vi "Main.vi"() -> ()   [LabVIEW 2014]
doc: "This template is for the Queued Message Handler design pattern.\n\nThe Event Handling Loop generates messages based on user interface actions.\n\nThe Message Handling Loop processes messages generated by the Event Handling Loop, or by other messages. The messages are string values, so new messages can be added easily to the Message Cases case structure in the Message Handling Loop. Each message cluster can also provide an optional value for Message Data, which is a variant that can be converted to whatever message-specific data is required."
uses:
  Support/Type Definitions/UI Data.ctl
  support/Message Queue/Message Queue.lvlib
  Support/User Event - EHL Stop/User Event - EHL Stop.lvlib
  Support/Message Queue/Enqueue Message (Single).vi
  <vilib>/ErrorRing/Error Ring.xnode
  Model/Model.lvlib
  PLC/PLC.lvlib
  Support/Status Logger/Status Log.ctl
  <vilib>/Utility/error.llb/Error Cluster From Error Code.vi
  Support/Global names.vi
panel:
  out "Power status":bool
  in  "Abort":bool
  in  "Stop Line":bool
  in  "Start Line":bool
  out "Status":string
  in  "Tab Control":enum32{"Simulation"}(tab)
  in  "Power switch":bool
  in  "Positon":dbl(slide) scale=0.0..20.0
  in  "Dispose":bool
  in  "Pump":bool
  in  "Flow [l/s]":dbl=10.0
  in  "Exit":bool
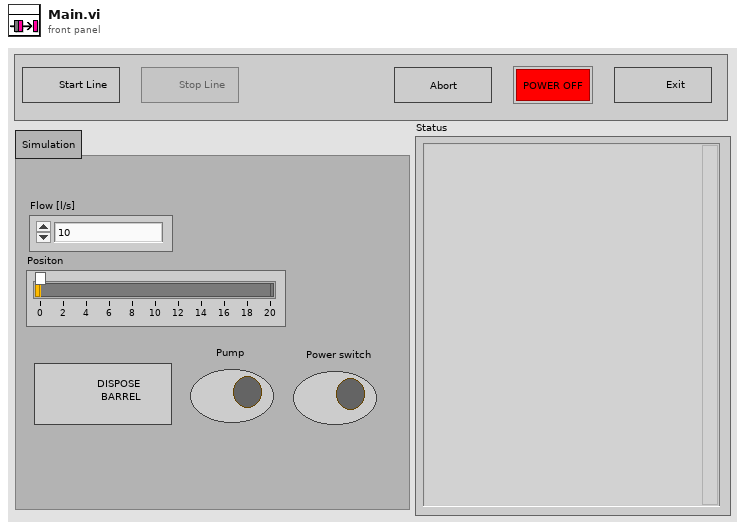
[diagram p1: front panel]
types:
  T1 = typedef "Status Log.ctl" = enum16{"Close file", "Open Status file", "Add Status", "Show Status File"}
  T2 = typedef "UI Data.ctl" = cluster{"Start Line Ref":refnum<vi>, "Stop Line Ref":refnum<vi>, "Data Display Ref":refnum<vi>, "Exit Button Ref":refnum<vi>, "Pump Ref":refnum<vi>, "Dispose Ref":refnum<vi>, "Flow Ref":refnum<vi>, "Position Ref":refnum<vi>, "Tab Ref":refnum<vi>, "Abort":refnum<vi>, "Power status":refnum<vi>, "Power switch":refnum<vi>}
  T3 = typedef "Notifiers.lvlib/Notifiers.ctl" = cluster{"PLC":refnum<notifier>, "Model":refnum<notifier>}
  T4 = typedef "Message Queue.lvlib/All Message Queues.ctl" = cluster{"UI":refnum<queue>, "Model":refnum<queue>, "PLC":refnum<queue>}
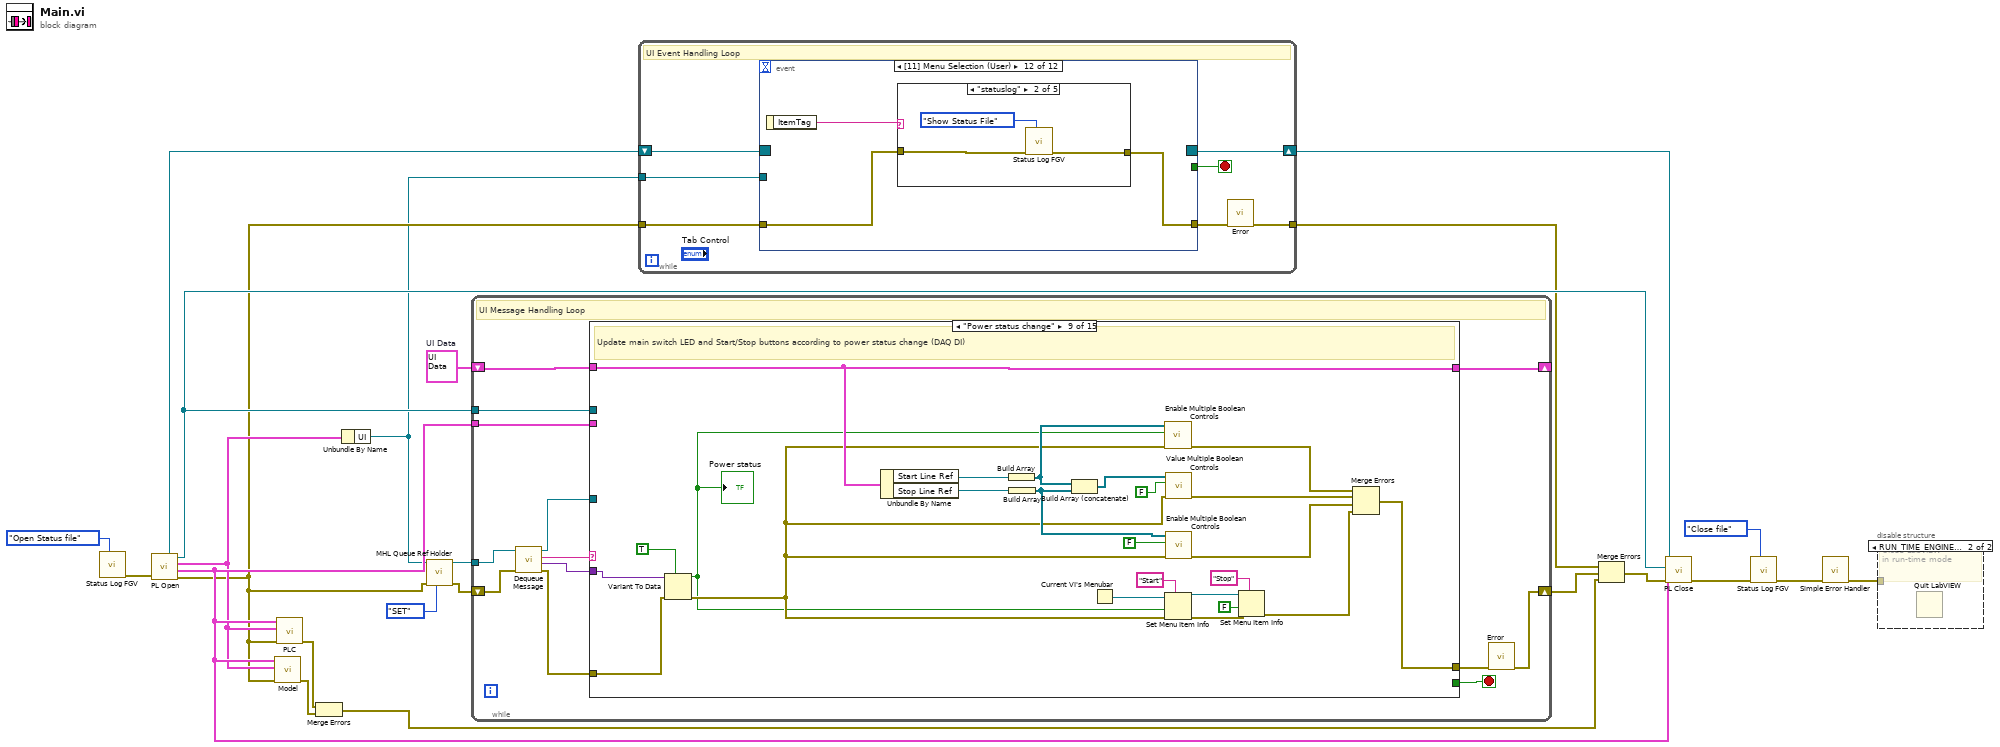
[diagram p0: block diagram]
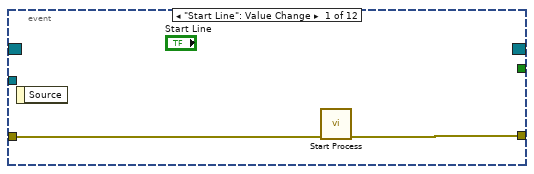
[diagram p2: hidden frame]
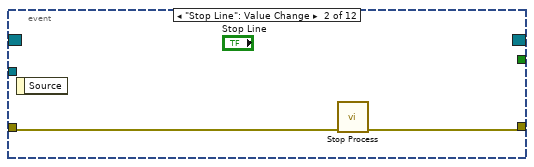
[diagram p3: hidden frame]
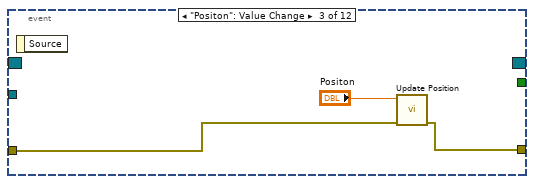
[diagram p4: hidden frame]
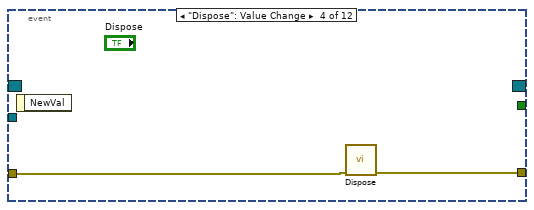
[diagram p5: hidden frame]
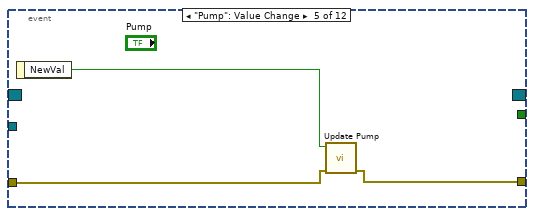
[diagram p6: hidden frame]
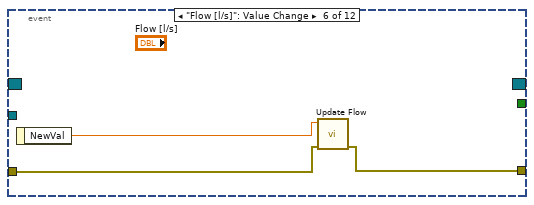
[diagram p7: hidden frame]
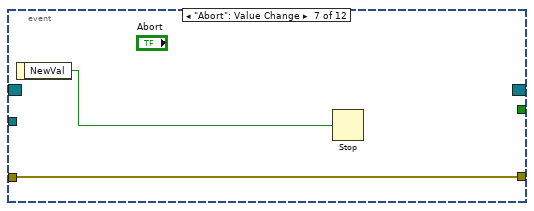
[diagram p8: hidden frame]
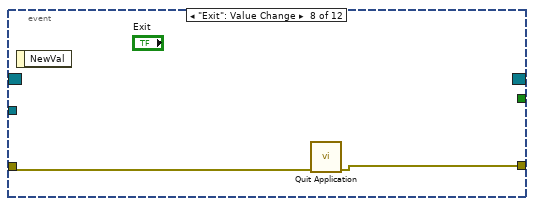
[diagram p9: hidden frame]
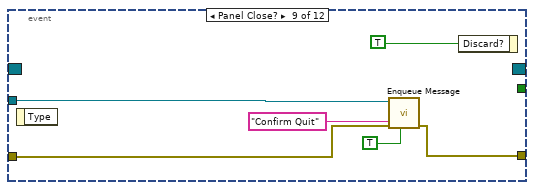
[diagram p10: hidden frame]
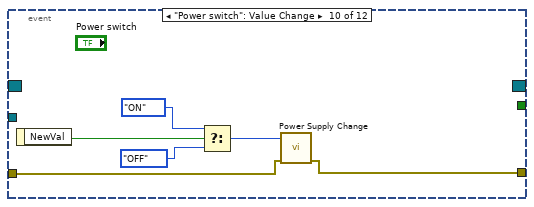
[diagram p11: hidden frame]
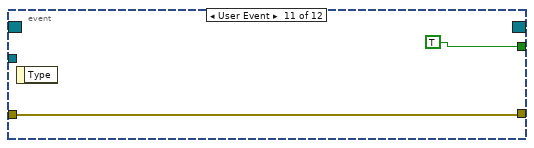
[diagram p12: hidden frame]
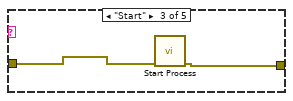
[diagram p14: hidden frame]
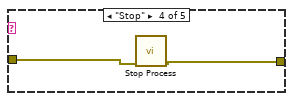
[diagram p15: hidden frame]
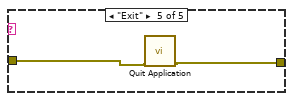
[diagram p16: hidden frame]
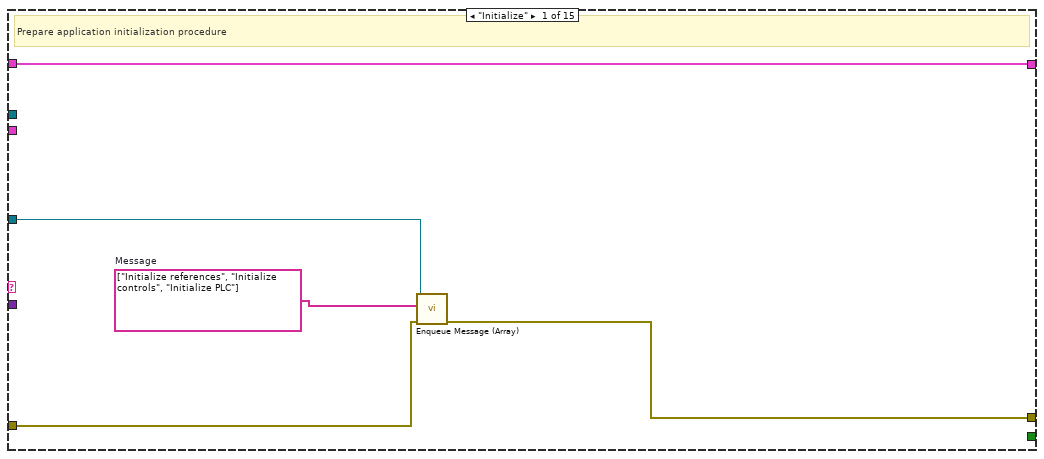
[diagram p18: hidden frame]
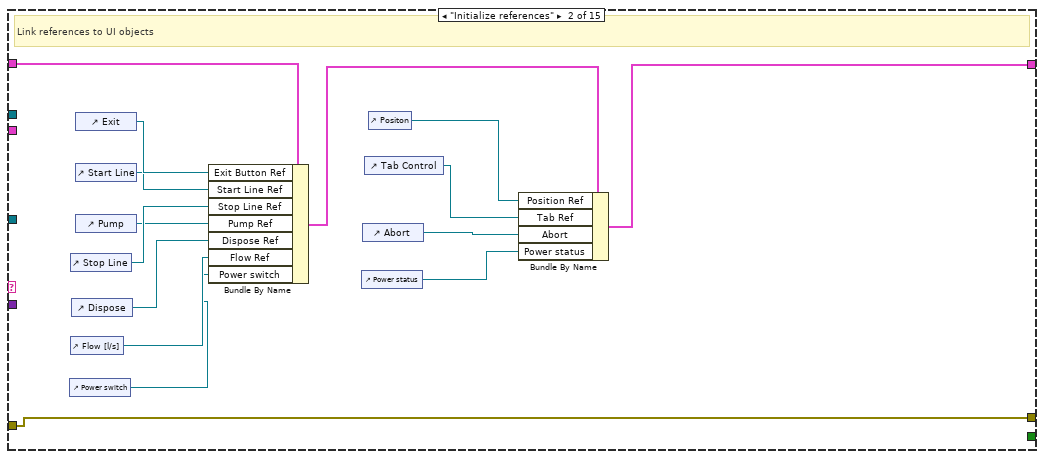
[diagram p19: hidden frame]
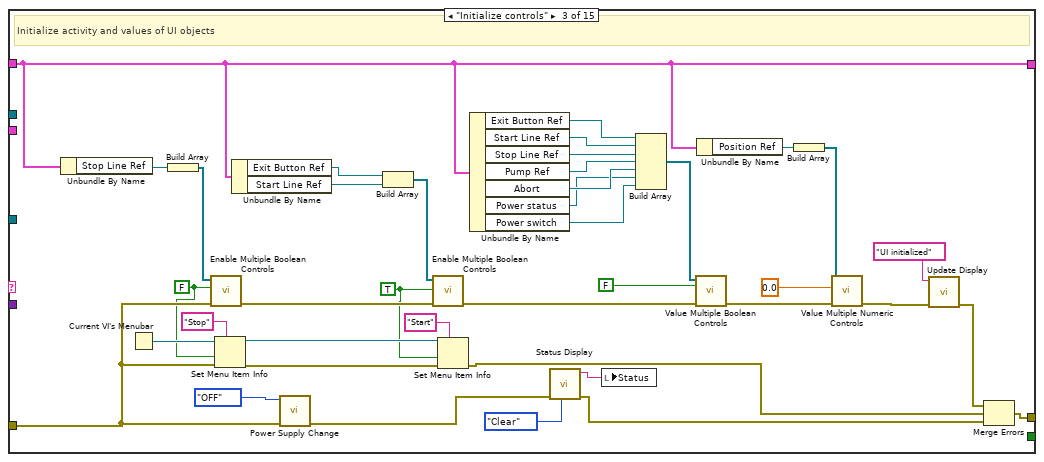
[diagram p20: hidden frame]
diagram:
  w22 = T2 {"Start Line Ref"=refnum, "Stop Line Ref"=refnum, "Data Display Ref"=refnum, "Exit Button Ref"=refnum, "Pump Ref"=refnum, "Dispose Ref"=refnum, "Flow Ref"=refnum, "Position Ref"=refnum, "Tab Ref"=refnum, "Abort"=refnum, "Power status"=refnum, "Power switch"=refnum}  # UI Data
  n1 = call "Status Log FGV.vi"("Action"=Status_Log."Open Status file") -> ("error out"=w17:errorcluster)  [unwired: 10 in]
  n2 = call "PL Open.vi"("error in"=w17) -> ("error out"=w4:errorcluster, "Notifiers"=w10:T3, "Queues"=w9:T4, "User Event"=w20:refnum<user-event>, "Event Registration Refnum"=w12:refnum<event-registration>)  [unwired: 6 in]
  n3 = call "Model.vi"("error in"=w4, "Queues"=w9, "Notifiers"=w10) -> ("error out"=w7:errorcluster)  [unwired: 8 in]
  n4 = call "PLC.vi"("error in"=w4, "Message Queues"=w9, "Notifiers"=w10) -> ("error out"=w8:errorcluster)  [unwired: 8 in]
  n5 = Merge Errors(w8, w7) -> (w6:errorcluster)
  n6 = Unbundle By Name(w9) -> ("UI"=w1:refnum<queue>)
  n7 = call "MHL Queue Ref Holder.vi"("Action"=enum16{"GET", "SET"}."SET", "error in"=w4, "Message Queue In"=w1) -> ("error out"=w3:errorcluster, "Input Message Queue"=w5:refnum<queue>)  [unwired: 7 in]
  n8 = while {
    shift-right: [w35] -> _
    shift-left: w22 -> [w36]
    tunnel: w20 -> [w33]
    tunnel: w10 -> [w29]
    shift-right: [w25] -> w16
    shift-left: w3 -> [w32]
    tunnel: w5 -> [w27]
    stop <- w34 stop-if-true
    # "UI Message Handling Loop"
    n9 = call "Dequeue Message.vi"("error in (no error)"=w32, "Message Queue"=w27) -> ("error out"=w31:errorcluster, "Message Data"=w28:variant, "Message"=w24:string, "dup Message Queue"=w30:refnum<queue>)  [unwired: 6 in]
    n10 = case "Message Cases" shown="\"Power status change\"" w24 {
      selector: w24 -> [_ _ _ _ _ _ _ _ _ _ _ _ _ _ w252]
      tunnel: w30 -> [w38 _ _ _ _ _ _ _ _ _ w198 w204 w240 _ _]
      tunnel: w31 -> [w39 w45 w65 w96 w112 w130 w143 w160 w188 w190 w199 w206 w223 w247 _]
      tunnel: [w37 w45 w74 w97 w111 w132 w145 w161 w182 w189 w196 w203 w227 w241 w251] -> w26
      tunnel: w36 -> [w40 w56 w82 w98 w117 w142 w151 w164 w185 w194 w200 w210 w232 w246 w253]
      tunnel: [w40 w46 w82 w98 w117 w142 w151 w164 w185 w194 w200 w210 w232 w246 w253] -> w35
      tunnel: [_ _ _ _ _ _ _ _ _ _ _ _ TRUE _ _] -> w34
      tunnel: w28 -> [_ _ _ _ _ _ w155 w158 w187 w193 _ _ w234 _ _]
      tunnel: w33 -> [_ _ _ _ _ _ _ _ _ _ _ _ w237 _ _]
      tunnel: w29 -> [_ _ _ _ _ _ _ _ _ _ _ w209 _ _ _]
      frame "Initialize" {
        w41 = string[] ["Initialize references", "Initialize controls", "Initialize PLC"]  # Message
        # "Prepare application initialization procedure"
        n11 = call "Enqueue Message (Array).vi"("error in (no error)"=w39, "Message Array"=w41, "Message Queue"=w38) -> ("error out"=w37:errorcluster)  [unwired: 7 in, 1 out]
      }
      frame "Initialize references" {
        # "Link references to UI objects"
        n12 = control-ref of="Power switch"() -> (w44:refnum<vi>)
        n13 = control-ref of="Stop Line"() -> (w53:refnum<vi>)
        n14 = control-ref of="Flow [l/s]"() -> (w50:refnum<vi>)
        n15 = control-ref of="Dispose"() -> (w51:refnum<vi>)
        n16 = control-ref of="Exit"() -> (w55:refnum<vi>)
        n17 = control-ref of="Start Line"() -> (w54:refnum<vi>)
        n18 = control-ref of="Pump"() -> (w52:refnum<vi>)
        n19 = Bundle By Name(cluster=w56, "Exit Button Ref"=w55, "Start Line Ref"=w54, "Stop Line Ref"=w53, "Pump Ref"=w52, "Dispose Ref"=w51, "Flow Ref"=w50, "Power switch"=w44) -> (w49:T2)
        n20 = control-ref of="Power status"() -> (w42:refnum<vi>)
        n21 = control-ref of="Abort"() -> (w43:refnum<vi>)
        n22 = control-ref of="Tab Control"() -> (w47:refnum<vi>)
        n23 = control-ref of="Positon"() -> (w48:refnum<vi>)
        n24 = Bundle By Name(cluster=w49, "Position Ref"=w48, "Tab Ref"=w47, "Abort"=w43, "Power status"=w42) -> (w46:T2)
      }
      frame "Initialize controls" {
        w57 = TRUE ("Enabled")
        w58 = FALSE ("Enabled")
        # "Initialize activity and values of UI objects"
        n25 = Unbundle By Name(w82) -> ("Stop Line Ref"=w95:refnum<vi>)
        n26 = Current VI's Menubar() -> (w60:refnum<k9>)
        n27 = Build Array(w95) -> (w94:refnum<vi>[])
        n28 = call "Enable Multiple Boolean Controls.vi"("error in"=w65, "Enabled"=w58, "References"=w94) -> ("error out"=w91:errorcluster)  [unwired: 8 in]
        n29 = Set Menu Item Info(7:"Stop" ("item tag"), 8:w65, 9:w58, 11:w60) -> (0:w63:errorcluster, 3:w59:refnum<k9>)  [unwired: 3 in]
        n30 = Unbundle By Name(w82) -> ("Exit Button Ref"=w93:refnum<vi>, "Start Line Ref"=w92:refnum<vi>)
        n31 = call "Power Supply Change.vi"("error in"=w65, "Power status"=enum16{"OFF", "ON"}."OFF") -> ("error out"=w71:errorcluster)  [unwired: 9 in]
        n32 = Build Array(w93, w92) -> (w90:refnum<vi>[])
        n33 = call "Enable Multiple Boolean Controls.vi"("error in"=w91, "Enabled"=w57, "References"=w90) -> ("error out"=w85:errorcluster)  [unwired: 8 in]
        n34 = Set Menu Item Info(7:"Start" ("item tag"), 8:w63, 9:w57, 11:w59) -> (0:w61:errorcluster)  [unwired: 3 in, 1 out]
        n35 = Unbundle By Name(w82) -> ("Exit Button Ref"=w89:refnum<vi>, "Start Line Ref"=w88:refnum<vi>, "Stop Line Ref"=w87:refnum<vi>, "Pump Ref"=w86:refnum<vi>, "Abort"=w77:refnum<vi>, "Power status"=w76:refnum<vi>, "Power switch"=w67:refnum<vi>)
        n36 = call "Status Display.vi"("Action"=enum16{"Update", "Clear"}."Clear", "error in"=w71) -> ("error out"=w70:errorcluster, "Status"=w68:string)  [unwired: 8 in]
        n37 = local write "Status"(w68) -> ()
        n38 = Build Array(w89, w88, w87, w86, w77, w76, w67) -> (w83:refnum<vi>[])
        n39 = call "Value Multiple Boolean Controls.vi"("error in"=w85, "Value"=FALSE ("Enabled"), "References"=w83) -> ("error out"=w81:errorcluster)  [unwired: 8 in]
        n40 = Unbundle By Name(w82) -> ("Position Ref"=w80:refnum<vi>)
        n41 = Build Array(w80) -> (w79:refnum<vi>[])
        n42 = call "Value Multiple Numeric Controls.vi"("error in"=w81, "Value"=0.0, "References"=w79) -> ("error out"=w73:errorcluster)  [unwired: 8 in]
        n43 = call "Update Display.vi"("error in"=w73, "Message string"="UI initialized") -> ("error out"=w62:errorcluster)  [unwired: 9 in]
        n44 = Merge Errors(w62, w61, w70) -> (w74:errorcluster)
      }
      frame "Initialize PLC" {
        # "Initialize Production Line Controller"
        n45 = call "Initialize.vi"("error in"=w96) -> ("error out"=w97:errorcluster)  [unwired: 10 in]
      }
      frame "Start process" {
        w103 = TRUE ("Enabled")
        w107 = FALSE ("Enabled")
        # "Starts process: start PLC, open logger file, create reports files, enable/disable UI controls and update status display"
        n46 = Unbundle By Name(w117) -> ("Exit Button Ref"=w100:refnum<vi>, "Start Line Ref"=w113:refnum<vi>, "Stop Line Ref"=w116:refnum<vi>)
        n47 = Build Array(w100, w113) -> (w118:refnum<vi>[])
        n48 = Build Array(w116) -> (w115:refnum<vi>[])
        n49 = call "Start.vi"("error in"=w112) -> ("error out"=w114:errorcluster)  [unwired: 10 in]
        n50 = call "Enable Multiple Boolean Controls.vi"("error in"=w112, "Enabled"=w103, "References"=w115) -> ("error out"=w105:errorcluster)  [unwired: 8 in]
        n51 = call "Enable Multiple Boolean Controls.vi"("error in"=w112, "Enabled"=w107, "References"=w118) -> ("error out"=w109:errorcluster)  [unwired: 8 in]
        n52 = global read "Global names.vi" "Starting"() -> (w101:string)
        n53 = Current VI's Menubar() -> (w102:refnum<k9>)
        n54 = call "Update Display.vi"("error in"=w114, "Message string"=w101) -> ("error out"=w99:errorcluster)  [unwired: 9 in]
        n55 = Set Menu Item Info(7:"Start" ("item tag"), 8:w109, 9:w107, 11:w102) -> (0:w108:errorcluster)  [unwired: 3 in, 1 out]
        n56 = Set Menu Item Info(7:"Stop" ("item tag"), 8:w105, 9:w103, 11:w102) -> (0:w104:errorcluster)  [unwired: 3 in, 1 out]
        n57 = Merge Errors(w99, w108, w104) -> (w111:errorcluster)
      }
      frame "Stop process" {
        w121 = FALSE ("Enabled")
        w122 = TRUE ("Enabled")
        # "Stops process: stop PLC, close logger file, save and close report files, enable/disable UI controls and update status display"
        n58 = Unbundle By Name(w142) -> ("Exit Button Ref"=w119:refnum<vi>, "Start Line Ref"=w135:refnum<vi>, "Stop Line Ref"=w141:refnum<vi>)
        n59 = call "Stop.vi"("error in"=w130) -> ("error out"=w137:errorcluster)  [unwired: 10 in]
        n60 = Build Array(w141) -> (w131:refnum<vi>[])
        n61 = Build Array(w119, w135) -> (w139:refnum<vi>[])
        n62 = global read "Global names.vi" "Stopping"() -> (w120:string)
        n63 = Build Array (concatenate)(w139, w131) -> (w138:refnum<vi>[])
        n64 = call "Enable Multiple Boolean Controls.vi"("error in"=w130, "Enabled"=w122, "References"=w139) -> ("error out"=w127:errorcluster)  [unwired: 8 in]
        n65 = call "Enable Multiple Boolean Controls.vi"("error in"=w130, "Enabled"=w121, "References"=w131) -> ("error out"=w134:errorcluster)  [unwired: 8 in]
        n66 = call "Value Multiple Boolean Controls.vi"("error in"=w130, "Value"=FALSE, "References"=w138) -> ("error out"=w133:errorcluster)  [unwired: 8 in]
        n67 = call "Update Display.vi"("error in"=w137, "Message string"=w120) -> ("error out"=w136:errorcluster)  [unwired: 9 in]
        n68 = Current VI's Menubar() -> (w128:refnum<k9>)
        n69 = Set Menu Item Info(7:"Start" ("item tag"), 8:w127, 9:w122, 11:w128) -> (0:w125:errorcluster, 3:w123:refnum<k9>)  [unwired: 3 in]
        n70 = Set Menu Item Info(7:"Stop" ("item tag"), 8:w125, 9:w121, 11:w123) -> (0:w124:errorcluster)  [unwired: 3 in, 1 out]
        n71 = Merge Errors(w136, w124, w134, w133) -> (w132:errorcluster)
      }
      frame "Update display" {
        # "Updates status display, status log file and word report file"
        n72 = Variant To Data(error in=w143, type="", Variant=w155) -> (data=w144:string, error out=w148:errorcluster)
        n73 = call "Status Display.vi"("Action"=enum16{"Update", "Clear"}."Update", "error in"=w148, "Status line"=w144) -> ("error out"=w146:errorcluster, "Status"=→"Status":string)  [unwired: 7 in]
        n74 = call "Status Log FGV.vi"("Action"=Status_Log."Add Status", "error in"=w148, "Status"=w144) -> ("error out"=w147:errorcluster)  [unwired: 8 in]
        n75 = property on="Status" class="Str"("Text.Scroll Position"=-1) -> ()  [unwired: 2 in, 2 out]
        n76 = Merge Errors(w143, w147, w146) -> (w145:errorcluster)
      }
      frame "Update position" {
        # "Programmatically update position of the barrel slider"
        n77 = Variant To Data(error in=w160, type=0.0 ("Value"), Variant=w158) -> (data=w156:dbl, error out=w159:errorcluster)
        n78 = Unbundle By Name(w164) -> ("Position Ref"=w163:refnum<vi>)
        n79 = Build Array(w163) -> (w162:refnum<vi>[])
        n80 = call "Value Multiple Numeric Controls.vi"("error in"=w159, "Value"=w156, "References"=w162) -> ("error out"=w161:errorcluster)  [unwired: 8 in]
      }
      frame "Power status change" {
        # "Update main switch LED and Start/Stop buttons according to power status change (DAQ DI)"
        n81 = Variant To Data(error in=w188, type=TRUE, Variant=w187) -> (data=w165:bool, error out=w169:errorcluster)
        "Power status" <- w165
        n82 = Unbundle By Name(w185) -> ("Start Line Ref"=w184:refnum<vi>, "Stop Line Ref"=w183:refnum<vi>)
        n83 = Build Array(w184) -> (w181:refnum<vi>[])
        n84 = Build Array(w183) -> (w178:refnum<vi>[])
        n85 = Build Array (concatenate)(w181, w178) -> (w180:refnum<vi>[])
        n86 = Current VI's Menubar() -> (w172:refnum<k9>)
        n87 = call "Enable Multiple Boolean Controls.vi"("error in"=w169, "Enabled"=w165, "References"=w181) -> ("error out"=w176:errorcluster)  [unwired: 8 in]
        n88 = Set Menu Item Info(7:"Start" ("item tag"), 8:w169, 9:w165, 11:w172) -> (0:w170:errorcluster, 3:w166:refnum<k9>)  [unwired: 3 in]
        n89 = call "Value Multiple Boolean Controls.vi"("error in"=w169, "Value"=FALSE, "References"=w180) -> ("error out"=w175:errorcluster)  [unwired: 8 in]
        n90 = call "Enable Multiple Boolean Controls.vi"("error in"=w169, "Enabled"=FALSE, "References"=w178) -> ("error out"=w174:errorcluster)  [unwired: 8 in]
        n91 = Set Menu Item Info(7:"Stop" ("item tag"), 8:w170, 9:FALSE ("enabled"), 11:w166) -> (0:w167:errorcluster)  [unwired: 3 in, 1 out]
        n92 = Merge Errors(w176, w175, w174, w167) -> (w182:errorcluster)
      }
      frame "Error" {
        # "Display error dialog box and quit application"
        n93 = Variant To Data(error in=w190, type=errorcluster {"status"=FALSE, "code"=0, "source"=""} ("error constant"), Variant=w193) -> (data=w191:errorcluster, error out=w189:errorcluster)
        n94 = call <vilib>:"Simple Error Handler.vi"("error in (no error)"=w191) -> ()  [unwired: 4 in, 5 out]
      }
      frame "Exit" {
        # "Start exit procedure: stop PLC, then send Exit message to PLC and go to PLC confirmation loop"
        n95 = Flush Queue(queue=w198, error in (no error)=w199) -> (error out=w195:errorcluster)  [unwired: 2 out]
        n96 = call "Exit PLC.vi"("error in"=w195) -> ("error out"=w197:errorcluster)  [unwired: 10 in]
        n97 = call "Wait on PLC Exit.vi"("error in"=w197) -> ("error out"=w196:errorcluster)  [unwired: 10 in]
      }
      frame "Wait on PLC exit" {
        # "Wait until PLC shutdown"
        n98 = Unbundle By Name(w209) -> ("PLC"=w208:refnum<notifier>)
        n99 = Wait on Notification(notifier=w208, timeout in ms (-1)=10, error in (no error)=w206) -> (notification=w202:string, timed out?=w205:bool, error out=w201:errorcluster)  [unwired: 1 in, 1 out]
        n100 = case shown="True" w205 {
          tunnel: [w211 w220] -> w203
          tunnel: w201 -> [w212 w217]
          tunnel: w204 -> [_ w218]
          tunnel: w202 -> [_ w213]
          frame True {
            # "Shutdown notification from PLC not received"
            n101 = call "Wait on PLC Exit.vi"("error in"=w212) -> ("error out"=w211:errorcluster)  [unwired: 10 in]
          }
          frame False {
            # "Shutdown notification from PLC received (handshake)"
            n102 = call "Update Display.vi"("error in"=w217, "Message string"=w213) -> ("error out"=w216:errorcluster)  [unwired: 9 in]
            n103 = call "Update Display.vi"("error in"=w216, "Message string"="Application quits" ("Message")) -> ("error out"=w215:errorcluster)  [unwired: 9 in]
            n104 = call-poly "Enqueue Message.vi"("error in (no error)"=w215, "Message"="End program", "Message Queue"=w218) -> ("error out"=w220:errorcluster)  [unwired: 7 in, 1 out]
          }
        }
      }
      frame "End program" {
        # "Shutdown MHL and send exit user event to EHL; reset UI controls"
        n105 = call "Fire User Event - EHL Stop.vi"("error in (no error)"=w223, "User Event - Stop"=w237) -> ("error out"=w222:errorcluster)  [unwired: 9 in]
        n106 = Variant To Data(error in=w223, type=errorcluster {"status"=FALSE, "code"=0, "source"=""} ("error constant"), Variant=w234) -> (data=w235:errorcluster)  [unwired: 1 out]
        n107 = Release Queue(queue=w240, force destroy? (F)=TRUE, error in (no error)=w223) -> (error out=w238:errorcluster)  [unwired: 2 out]
        n108 = call <vilib>:"Simple Error Handler.vi"("error in (no error)"=w235) -> ("error out"=w221:errorcluster)  [unwired: 4 in, 4 out]
        n109 = Merge Errors(w222, w221, w238) -> (w228:errorcluster)
        n110 = Unbundle By Name(w232) -> ("Exit Button Ref"=w231:refnum<vi>, "Abort"=w226:refnum<vi>, "Start Line Ref"=w225:refnum<vi>, "Stop Line Ref"=w224:refnum<vi>)
        n111 = Build Array(w231, w226, w225, w224) -> (w230:refnum<vi>[])
        n112 = call "Value Multiple Boolean Controls.vi"("error in"=w228, "Value"=FALSE, "References"=w230) -> ("error out"=w227:errorcluster)  [unwired: 8 in]
      }
      frame "Confirm Quit" {
        # "Confirm Quit - Message that can confirm whether or not the user wants to exit the application."
        n113 = Two Button Dialog(message="Are you sure?", 1:"Continue" ("F button name (\"Cancel\")"), 2:"Quit" ("T button name (\"OK\")")) -> (T button?=w242:bool)
        n114 = case shown="True" w242 {
          tunnel: w247 -> [w248 w250]
          tunnel: [w248 w249] -> w241
          frame False {
          }
          frame True {
            n115 = call "Quit Application.vi"("error in"=w250) -> ("error out"=w249:errorcluster)  [unwired: 10 in]
          }
        }
      }
      frame Default {
        # "Incorrect message: show error and clear error"
        n116 = xnode "Error Ring"("parameter 0"=w252) -> ("error out"=w251:errorcluster)
      }
    }
    n117 = call "Error.vi"("error in"=w26) -> ("error out"=w25:errorcluster)  [unwired: 10 in]
  }
  n118 = while {
    tunnel: w1 -> [w263]
    shift-right: [w266] -> w23
    shift-left: w12 -> [w267]
    tunnel: [w261] -> w11
    tunnel: w4 -> [w264]
    stop <- w265 stop-if-true
    # "UI Event Handling Loop"
    n119 = event shown="[11] Menu Selection (User)" {
      selector: w267 -> [_ _ _ _ _ _ _ _ _ _ _ _]
      dyn-events: [_ _ _ _ _ _ _ _ _ _ _ _] -> w266
      timeout: _ -> [_ _ _ _ _ _ _ _ _ _ _ _]
      tunnel: [_ _ _ _ _ _ _ _ _ _ TRUE ("Discard?") _] -> w265
      tunnel: w263 -> [_ _ _ _ _ _ _ _ w292 _ _ _]
      tunnel: [w268 w270 w273 w275 w278 w281 w284 w285 w291 w293 w299 w302] -> w262
      tunnel: w264 -> [w269 w271 w272 w276 w279 w282 w284 w286 w287 w294 w299 w301]
      event "Start Line": Value Change {
        n120 = event-data() -> ()  [unwired: 1 in, 1 out]
        n121 = call "Start Process.vi"("error in"=w269) -> ("error out"=w268:errorcluster)  [unwired: 10 in]
      }
      event "Stop Line": Value Change {
        n122 = event-data() -> ()  [unwired: 1 in, 1 out]
        n123 = call "Stop Process.vi"("error in"=w271) -> ("error out"=w270:errorcluster)  [unwired: 10 in]
      }
      event "Positon": Value Change {
        n124 = event-data() -> ()  [unwired: 1 in, 1 out]
        n125 = call "Update Position.vi"("error in (no error)"=w272, "Position"="Positon") -> ("error out"=w273:errorcluster)  [unwired: 9 in]
      }
      event "Dispose": Value Change {
        n126 = event-data() -> ()  [unwired: 1 in, 1 out]
        n127 = call "Dispose.vi"("error in (no error)"=w276) -> ("error out"=w275:errorcluster)  [unwired: 10 in]
      }
      event "Pump": Value Change {
        n128 = event-data() -> ("NewVal"=w277:bool)  [unwired: 1 in]
        n129 = call "Update Pump.vi"("error in (no error)"=w279, "Pump State"=w277) -> ("error out"=w278:errorcluster)  [unwired: 9 in]
      }
      event "Flow [l/s]": Value Change {
        n130 = event-data() -> ("NewVal"=w280:dbl)  [unwired: 1 in]
        n131 = call "Update Flow.vi"("error in (no error)"=w282, "Flow"=w280) -> ("error out"=w281:errorcluster)  [unwired: 9 in]
      }
      event "Abort": Value Change {
        n132 = event-data() -> ("NewVal"=w283:bool)  [unwired: 1 in]
        n133 = Stop(stop? (T)=w283) -> ()
      }
      event "Exit": Value Change {
        n134 = event-data() -> ()  [unwired: 1 in, 1 out]
        n135 = call "Quit Application.vi"("error in"=w286) -> ("error out"=w285:errorcluster)  [unwired: 10 in]
      }
      event Panel Close? {
        n136 = event-data() -> ()  [unwired: 1 in, 1 out]
        n137 = call-poly "Enqueue Message.vi"("Priority Message? (F)"=TRUE, "error in (no error)"=w287, "Message"="Confirm Quit", "Message Queue"=w292) -> ("error out"=w291:errorcluster)  [unwired: 6 in, 1 out]
        n138 = event-data("Discard?"=TRUE) -> ()  [unwired: 1 in, 1 out]
      }
      event "Power switch": Value Change {
        n139 = event-data() -> ("NewVal"=w298:bool)  [unwired: 1 in]
        n140 = Select(t=enum16{"OFF", "ON"}."ON" ("Power status"), s=w298, f=enum16{"OFF", "ON"}."OFF" ("Power status")) -> (s? t:f=w295:enum16{"OFF", "ON"})
        n141 = call "Power Supply Change.vi"("error in"=w294, "Power status"=w295) -> ("error out"=w293:errorcluster)  [unwired: 9 in]
      }
      event User Event {
        n142 = event-data() -> ()  [unwired: 1 in, 1 out]
      }
      event Menu Selection (User) {
        n143 = event-data() -> ("ItemTag"=w303:string)  [unwired: 1 in]
        n144 = case shown="\"statuslog\"" w303 {
          tunnel: [w304 w305 w309 w310 w312] -> w302
          tunnel: w301 -> [w304 w306 w308 w311 w313]
          frame Default {
          }
          frame "statuslog" {
            n145 = call "Status Log FGV.vi"("Action"=Status_Log."Show Status File", "error in"=w306) -> ("error out"=w305:errorcluster)  [unwired: 9 in]
          }
          frame "Start" {
            n146 = call "Start Process.vi"("error in"=w308) -> ("error out"=w309:errorcluster)  [unwired: 10 in]
          }
          frame "Stop" {
            n147 = call "Stop Process.vi"("error in"=w311) -> ("error out"=w310:errorcluster)  [unwired: 10 in]
          }
          frame "Exit" {
            n148 = call "Quit Application.vi"("error in"=w313) -> ("error out"=w312:errorcluster)  [unwired: 10 in]
          }
        }
      }
    }
    n149 = call "Error.vi"("error in"=w262) -> ("error out"=w261:errorcluster)  [unwired: 10 in]
  }
  n150 = Merge Errors(w11, w16, w6) -> (w15:errorcluster)
  n151 = call "PL Close.vi"("error in"=w15, "Notifiers"=w10, "User Event"=w20, "Event Registration Refnum in"=w23) -> ("error out"=w21:errorcluster)  [unwired: 7 in]
  n152 = call "Status Log FGV.vi"("Action"=Status_Log."Close file", "error in"=w21) -> ("error out"=w13:errorcluster)  [unwired: 9 in]
  n153 = call <vilib>:"Simple Error Handler.vi"("error in (no error)"=w13) -> ("error out"=w14:errorcluster)  [unwired: 4 in, 4 out]
  n154 = disable-structure shown="RUN_TIME_ENGINE==True" {
    disable-tunnel: w14 -> [_ _]
    frame condition #0 (active) {
    }
    frame condition #1 {
      # "Close LabVIEW\nin run-time mode"
      n155 = Quit LabVIEW() -> ()  [unwired: 1 in]
    }
  }
